vi "Creador_Arreglo.vi"() -> ()   [LabVIEW 2016]
uses:
  <vilib>/imath/engines/lvmath2/RunTimeEngine/RangeToken/NIMS_Range_R3 - Integer.vi
  <instcachedir>/0/NIMS_Range_R3 - Integer_A435E2FF893B4C718FD5055FE39FE2F6.lvgen/NIMS_Range_R3 - Integer_A435E2FF893B4C718FD5055FE39FE2F6_000.vi
  <vilib>/imath/engines/lvmath2/RunTimeEngine/CommandStatement/MC_CommandStatement_break.vi
  <vilib>/imath/engines/lvmath2/RunTimeEngine/VariableToken/NIMS_VariableToken_CondDefinedDefinedByReplace.vi
  <instcachedir>/0/NIMS_VariableToken_CondDefinedDefinedByReplace_D162CFFC24174562A9FEA619A91E1A56.lvgen/NIMS_VariableToken_CondDefinedDefinedByReplace_D162CFFC24174562A9FEA619A91E1A56_001.vi
  <vilib>/imath/engines/lvmath2/RunTimeEngine/BuiltInFunctions/round/NIMS_round(DBL-S).vi
  <vilib>/imath/engines/lvmath2/RunTimeEngine/IndexReplace/NIMS M(S,S)=S.vi
  <instcachedir>/0/NIMS M(S,S)=S_98E40400474E4398B113AE20298B4F82.lvgen/NIMS M(S,S)=S_98E40400474E4398B113AE20298B4F82_000.vi
  <vilib>/imathl/engines/lvmath/Functions/Error Handling/Create Error.vi
  <vilib>/imath/engines/lvmath2/RunTimeEngine/VariableToken/NIMS_VariableToken_CondDefined.vi
  <instcachedir>/0/NIMS_VariableToken_CondDefined_06E9DA95BD4D46A6BA55EC651A891960.lvgen/NIMS_VariableToken_CondDefined_06E9DA95BD4D46A6BA55EC651A891960_001.vi
  <vilib>/imath/engines/lvmath/Functions/Error Handling/MergeErrorsWrapper.vi
  <vilib>/imath/engines/lvmath2/RunTimeEngine/NodeEndStatement/NIMS_NodeEndStatement_Output.vi
  <instcachedir>/0/NIMS_NodeEndStatement_Output_53EC0D466D134D7ABD903AC30B43404B.lvgen/NIMS_NodeEndStatement_Output_53EC0D466D134D7ABD903AC30B43404B_012.vi
  <vilib>/imath/engines/lvmath2/RunTimeEngine/ErrorHandling/NIMS_Finalize Error.vi
panel:
  out "Numeric Control":i32
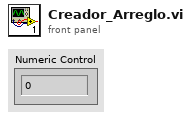
[diagram p1: front panel]
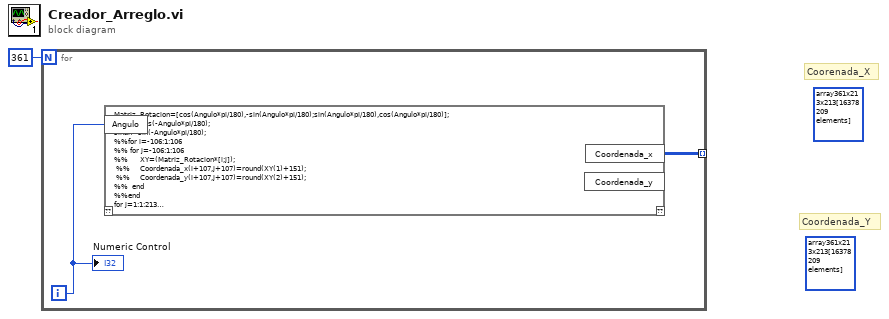
[diagram p0: block diagram]
diagram:
  (unwired) i16[][][] array361x213x213[16378209 elements] ("Coordenada_y")
  (unwired) i16[][][] array361x213x213[16378209 elements] ("Coordenada_x")
  # "Coorenada_X"
  # "Coordenada_Y"
  n1 = for {
    N: 361 -> [_]
    tunnel: [w2] -> _ mode=indexing
    i -> [w3]
    n2 = mathscript code="Matriz_Rotacion=[cos(Angulo*pi/180),-sin(Angulo*pi/180);sin(Angulo*pi/180),cos(Angulo*pi/180)];\ncosan=cos(-Angulo*pi/180);\nsinan=sin(-Angulo*pi/180);\n%%for i=-106:1:106\n%% for j=-106:1:106\n%%      XY=(Matriz_Rotacion*[i;j]);\n %%     Coordenada_x(i+107,j+107)=round(XY(1)+151);\n %%     Coordenada_y(i+107,j+107)=round(XY(2)+151);\n%%  end\n%%end\nfor j=1:1:213\n for i=1:1:213\n       Coordenada_x(i,j)=round((i-107)*cosan-(j-107)*sinan+151);\n       Coordenada_y(i,j)=round((i-107)*sinan+(j-107)*cosan+151);\n end\nend"("Angulo"=w3) -> ("Coordenada_x"=w2:i16[][])  [unwired: 1 in, 2 out]
    "Numeric Control" <- w3
  }
